vi "Search and Split String.vi"(1 "String 2":string) -> (0 "String":string)   [LabVIEW 2010]
panel:
  in  "offset (0)":i32
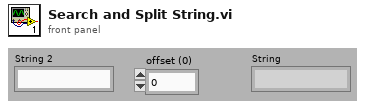
[diagram p1: front panel]
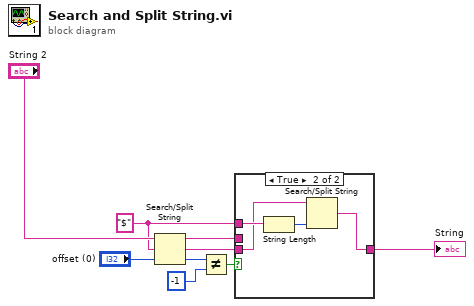
[diagram p0: block diagram]
diagram:
  w1 = "$" ("search string/char (-)")
  n1 = Search/Split String(string="String 2", search string/char (-)=w1, offset (0)="offset (0)") -> (substring before match=w6:string, match + rest of string=w5:string, offset of match=w2:i32)
  n2 = Not Equal?(x=w2, y=-1) -> (x != y?=w3:bool)
  n3 = case "Trim Match from Rest of String?" shown="True" w3 {
    tunnel: w1 -> [_ w14]
    tunnel: w6 -> [_ _]
    tunnel: w5 -> [w10 w13]
    tunnel: [w10 w11] -> w9
    frame False {
    }
    frame True {
      n4 = String Length(string=w14) -> (length=w12:i32)
      n5 = Search/Split String(string=w13, offset (0)=w12) -> (match + rest of string=w11:string)  [unwired: 1 in, 2 out]
    }
  }
  "String" <- w9
